vi "CrsrList to MaxMin.vi"(11 "CrsrList":T1) -> (2 "Min":dbl, 3 "Max":dbl)   [LabVIEW 2012]
uses:
  <vilib>/Utility/miscctls.llb/LVCursorListTypeDef.ctl
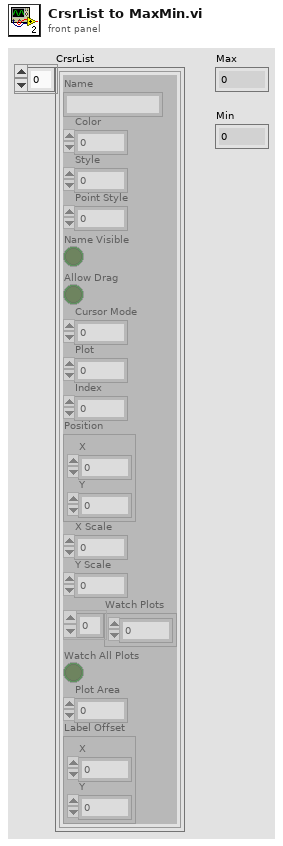
[diagram p1: front panel]
types:
  T1 = typedef "LVCursorListTypeDef.ctl" = cluster{"Name":string, "Color":u32, "Style":u8, "Point Style":u8, "Name Visible":bool, "Allow Drag":bool, "Cursor Mode":u32, "Plot":i32, "Index":i32, "Position":cluster{"X":dbl, "Y":dbl}, "X Scale":u32, "Y Scale":u32, "Watch Plots":i32[], "Watch All Plots":bool, "Plot Area":i32, "Label Offset":cluster{"X":dbl, "Y":dbl}}[]
  T2 = cluster{"Name":string, "Color":u32, "Style":u8, "Point Style":u8, "Name Visible":bool, "Allow Drag":bool, "Cursor Mode":u32, "Plot":i32, "Index":i32, "Position":cluster{"X":dbl, "Y":dbl}, "X Scale":u32, "Y Scale":u32, "Watch Plots":i32[], "Watch All Plots":bool, "Plot Area":i32, "Label Offset":cluster{"X":dbl, "Y":dbl}}
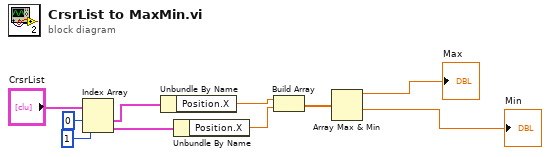
[diagram p0: block diagram]
diagram:
  n1 = Index Array(array="CrsrList", index #1=0 ("index"), index #2=1 ("index")) -> (element #1=w3:T2, element #2=w5:T2)
  n2 = Unbundle By Name(w3) -> ("Position.X"=w6:dbl)
  n3 = Unbundle By Name(w5) -> ("Position.X"=w7:dbl)
  n4 = Build Array(w6, w7) -> (w8:dbl[])
  n5 = Array Max & Min(array=w8) -> (max value=→"Max":dbl, min value=→"Min":dbl)  [unwired: 2 out]
